vi "Enable Inputs.vi"(8 "error in (no error)":errorcluster, 9 "Enable Input (F: False)":bool, 10 "Enable Remote Sense (F: False)":bool, 11 "VISA resource name":refnum<visa-resource-name>) -> (0 "error out":errorcluster, 3 "VISA resource name out":refnum<visa-resource-name>)   [LabVIEW 2020, in "BK Precision 8600 Series.lvlib"]
doc: "Enables or disables input state and controls the state of remote sense."
uses:
  BK Precision 8600 Series.lvlib
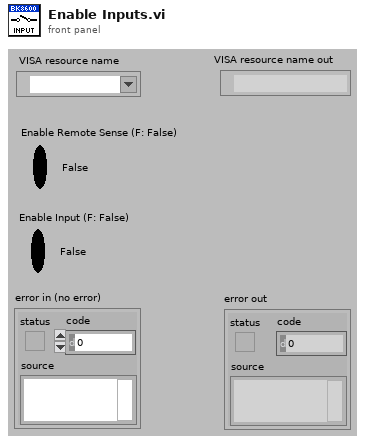
[diagram p1: front panel]
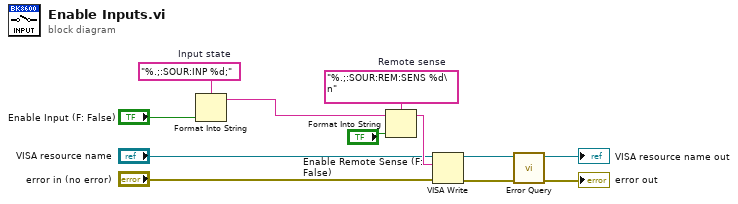
[diagram p0: block diagram]
diagram:
  w6 = "%.;:SOUR:REM:SENS %d\n"  # Remote sense
  w7 = "%.;:SOUR:INP %d;"  # Input state
  n1 = Format Into String(format string=w7, "Enable Input (F: False)") -> (resulting string=w4:string)  [unwired: 2 in, 1 out]
  n2 = Format Into String(format string=w6, initial string=w4, "Enable Remote Sense (F: False)") -> (resulting string=w3:string)  [unwired: 1 in, 1 out]
  n3 = VISA Write(VISA resource name="VISA resource name", write buffer=w3, error in (no error)="error in (no error)") -> (VISA resource name out=w9:refnum<visa-resource-name>, error out=w8:errorcluster)  [unwired: 1 out]
  n4 = call "Error Query.vi"("error in (no error)"=w8, "VISA resource name"=w9) -> ("error out"=→"error out":errorcluster, "VISA resource name out"=→"VISA resource name out":refnum<visa-resource-name>)  [unwired: 6 in, 2 out]
